vi "GEA2 Send and Receive Message.vi"(0 "GEA2 Reference In":refnum<k24>, 1 "Input Data":T1 {"Command" format="%02x"; "Destination" format="%02x"; "Source" format="%02x"}, 2 "Read Timeout (ms)":u32=500, 5 "Expected Command":string=".*", 7 "Expected Data":string=".*", 9 "Expected Data 2":string, 11 "Error In":errorcluster, 13 "Expected Command 2":string=".*", 14 "Disable Expected Data":bool) -> (4 "GEA2 Reference Out":refnum<k24>, 6 "Raw Data Out":string, 8 "Converted Data Out":T2 {"CRC" format="%04x"; "Length" format="%02x"; "Command" format="%02x"; "Destination" format="%02x"; "Source" format="%02x"}, 15 "Error Out":errorcluster)   [LabVIEW 2014, in "GEA2_Toolkit.lvlib"]
doc: "This VI sends and receives data across the GEA2 bus. The VI waits for the expected responses (filtered by the expected command / data fields) or until the timeout occurs."
uses:
  library/GEA2_Toolkit.lvlib
  type defs/Data Out.ctl
  type defs/Data In.ctl
  C:/Automation/DLLs/PC Tools .NET/GeaCommunication.dll
  Automation/DLLs/PC Tools .NET/GeaCommunication.dll
panel:
  out "error IO":errorcluster
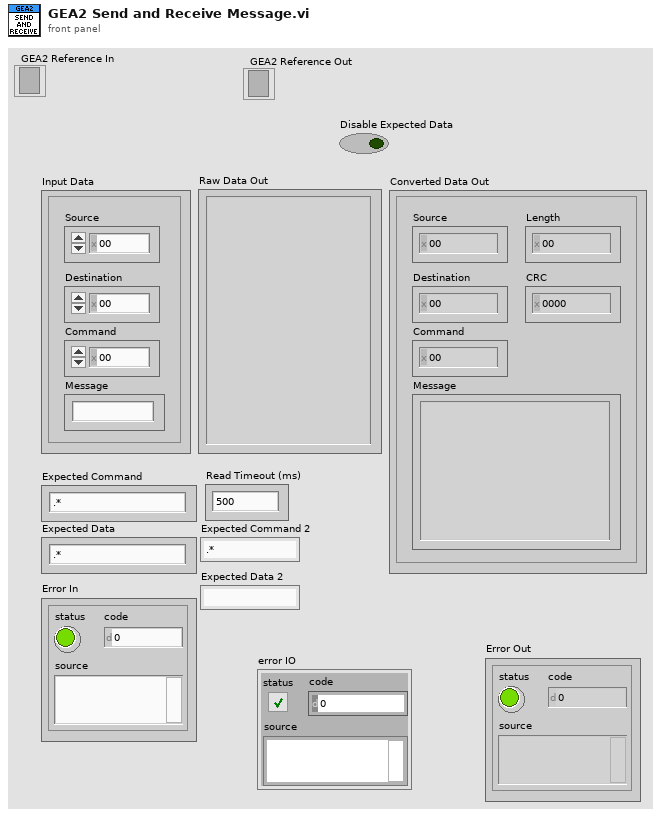
[diagram p1: front panel]
types:
  T1 = typedef "GEA2_Toolkit.lvlib/Data In.ctl" = cluster{"Source":u8, "Destination":u8, "Command":u8, "Message":string}
  T2 = typedef "GEA2_Toolkit.lvlib/Data Out.ctl" = cluster{"Source":u8, "Destination":u8, "Command":u8, "Length":u8, "CRC":u16, "Message":string}
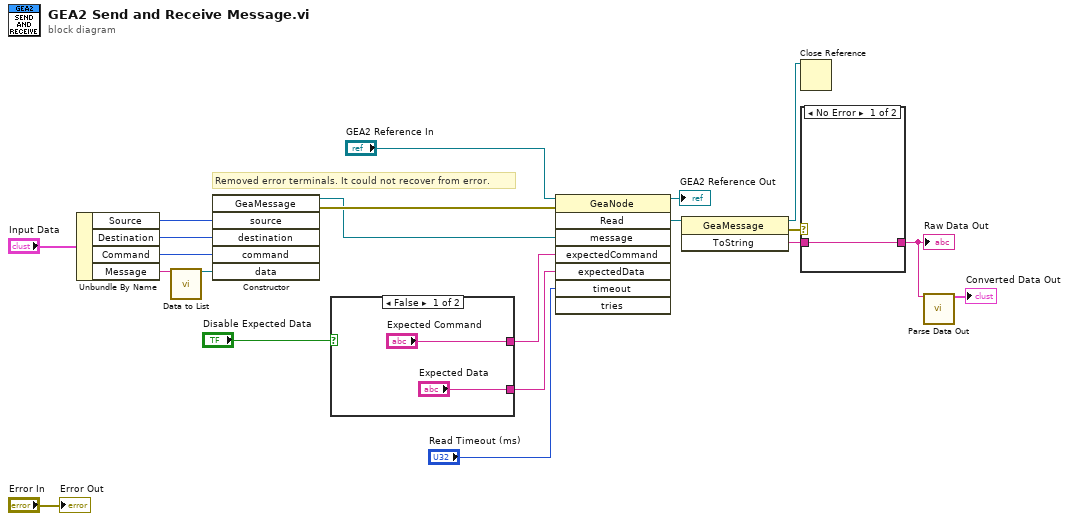
[diagram p0: block diagram]
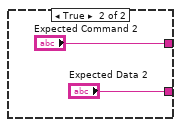
[diagram p2: hidden frame]
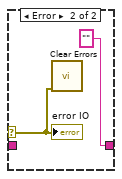
[diagram p3: hidden frame]
diagram:
  # "Removed error terminals. It could not recover from error."
  n1 = Unbundle By Name("Input Data") -> ("Source"=w10:u8, "Destination"=w11:u8, "Command"=w12:u8, "Message"=w13:string)
  n2 = call "Data to List.vi"("Data String In"=w13) -> ("GEA List"=w1:refnum<k24>)  [unwired: 13 in, 1 out]
  n3 = constructor class="GeaMessage"("source"=w10, "destination"=w11, "command"=w12, "data"=w1) -> (reference out=w4:refnum<k24>, error out=w5:errorcluster)  [unwired: 3 in, 5 out]
  n4 = case shown="False" "Disable Expected Data" {
    tunnel: ["Expected Data" "Expected Data 2"] -> w8
    tunnel: ["Expected Command" "Expected Command 2"] -> w7
    frame False {
    }
    frame True {
    }
  }
  n5 = invoke class="GeaNode" method="Read"(reference="GEA2 Reference In", error in=w5, "message"=w4, "expectedCommand"=w7, "expectedData"=w8, "timeout"="Read Timeout (ms)") -> (reference out=→"GEA2 Reference Out":refnum<k24>, "Read"=w14:refnum<k24>)  [unwired: 2 in, 6 out]
  n6 = invoke class="GeaMessage" method="ToString"(reference=w14) -> (reference out=w15:refnum<k24>, error out=w6:errorcluster, "ToString"=w16:string)  [unwired: 2 in]
  n7 = Close Reference(reference=w15) -> ()  [unwired: 1 in, 1 out]
  n8 = case shown="No Error" w6 {
    selector: w6 -> [_ w27]
    tunnel: w16 -> [w26 _]
    tunnel: [w26 "" ("ToString")] -> w21
    frame No Error {
    }
    frame Error {
      n9 = call <vilib>:"Clear Errors.vi"("error in (no error)"=w27) -> ()  [unwired: 5 in, 2 out]
      "error IO" <- w27
    }
  }
  "Raw Data Out" <- w21
  n10 = call "Parse Data Out.vi"("Raw Data In"=w21) -> ("Data Out"=→"Converted Data Out":T2)  [unwired: 13 in, 1 out]
  "Error Out" <- "Error In"
